vi "subvi4.vi"(8 "error in (no error)":errorcluster, 9 "Motor Step/Direction":u16, 10 "Speed":u32, 11 "Refnum in":refnum<k21>) -> (0 "error out":errorcluster, 2 "Numeric":dbl, 3 "Refnum out":refnum<k21>)   [LabVIEW 2018]
uses:
  <vilib>/DAQmx/write.llb/DAQmx Write (Digital U8 1Chan 1Samp).vi
  <vilib>/DAQmx/miscellaneous.llb/DAQmx Fill In Error Info.vi
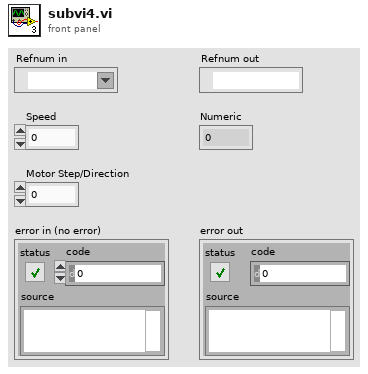
[diagram p1: front panel]
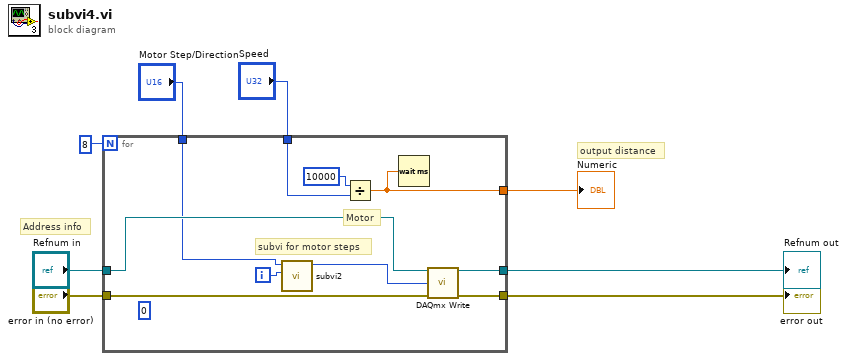
[diagram p0: block diagram]
diagram:
  # "output distance"
  # "Address info"
  n1 = for {
    N: 8 -> [_]
    tunnel: "error in (no error)" -> [w16]
    tunnel: "Refnum in" -> [w15]
    tunnel: [w13] -> w4
    tunnel: [w12] -> w5
    tunnel: [w11] -> w6
    tunnel: "Speed" -> [w10]
    tunnel: "Motor Step/Direction" -> [w9]
    i -> [w18]
    (unwired) 0
    # "subvi for motor steps"
    # "Motor"
    n2 = call "subvi2.vi"("Numeric in"=w18, "Motor Step/Direction"=w9) -> ("Numeric out"=w17:u32)  [unwired: 9 in]
    n3 = Divide(x=u32 10000, y=w10) -> (x/y=w13:dbl)
    n4 = Wait (ms)(milliseconds to wait=w13) -> ()  [unwired: 1 out]
    n5 = call-poly <vilib>:"DAQmx Write.vi"("task/channels in"=w15, "data"=w17, "error in"=w16) -> ("task out"=w11:refnum<k21>, "error out"=w12:errorcluster)  [unwired: 10 in, 1 out]
  }
  "Refnum out" <- w6
  "error out" <- w5
  "Numeric" <- w4
